vi "step_set_hipot_hold_time.vi"(8 "error in":errorcluster, 10 "step":T3 {"data num" format="%.3f"}) -> (0 "error out":errorcluster, 2 "test results":T1)   [LabVIEW 2020]
uses:
  controls/PROTO_stepV2.ctl
  controls/step_type.ctl
  controls/test results.ctl
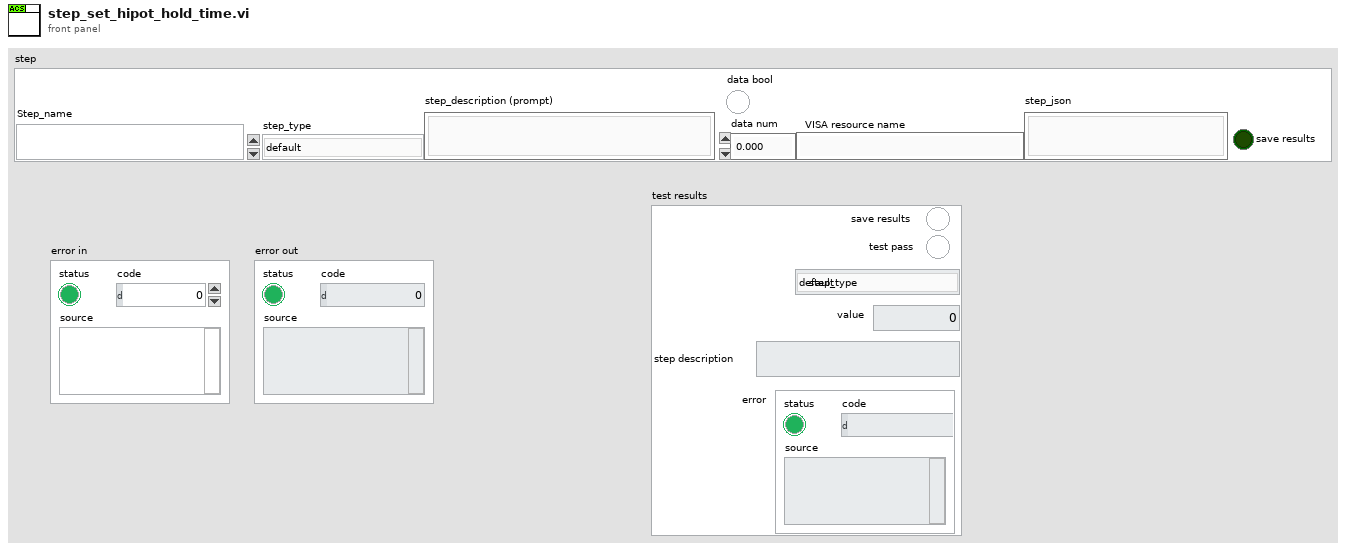
[diagram p1: front panel]
types:
  T1 = typedef "test results.ctl" = cluster{"test pass":bool, "step_type":T2, "value":dbl, "step description":string, "error":errorcluster, "save results":bool}
  T2 = typedef "step_type.ctl" = enum16{"default", "prompt", "sequence#", "12V_1_power supply on_off", "12V_2_power supply on_off", "set_hipot_V", "set_hipot_I_limit", "set_hipot_ramping (sec)", "set hipot_hold_time", "read_hipot_V", "read_hipot_I", "set_daq", "read_daq", "flash uds", "wait (sec)", "record_pass_fail", "ac_charge_test", "dc_400V_charging", "HAPS Heater Output", "HAPS Compressor Output", "stop_test", "error_exit"}
  T3 = typedef "PROTO_stepV2.ctl" = cluster{"VISA resource name":string, "data num":dbl, "step_description (prompt)":string, "step_json":string, "save results":bool, "step_type":T2, "Step_name":string, "data bool":bool}
  T4 = cluster{"error":bool, "code":i8, "source":string}
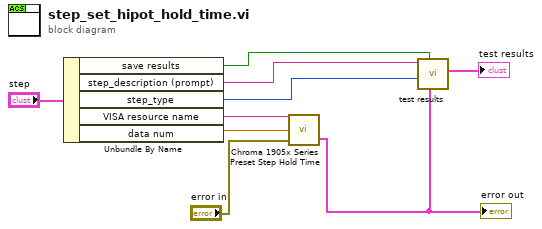
[diagram p0: block diagram]
diagram:
  n1 = Unbundle By Name("step") -> ("save results"=w1:bool, "step_description (prompt)"=w2:string, "step_type"=w3:T2, "VISA resource name"=w8:string, "data num"=w9:dbl)
  n2 = call <instrlib>:"Chroma 1905x Series Preset Step Hold Time.vi"("error in"="error in", "Step Time"=w9, "inst handle in"=w8) -> ("error out"=w4:T4)  [unwired: 1 out]
  "error out" <- w4
  n3 = call "test results.vi"("error"=w4, "save results"=w1, "step_type"=w3, "(description) used in test"=w2) -> ("test results"=→"test results":T1)  [unwired: 7 in]
